vi "init.vi"(10 "WebBrowser":refnum<k7>(container), 11 "VI in":refnum<vi>) -> (0 "error out":errorcluster, 1 "Lab Description:":string, 2 "solution":dbl, 3 "lab":dbl)   [LabVIEW 2014]
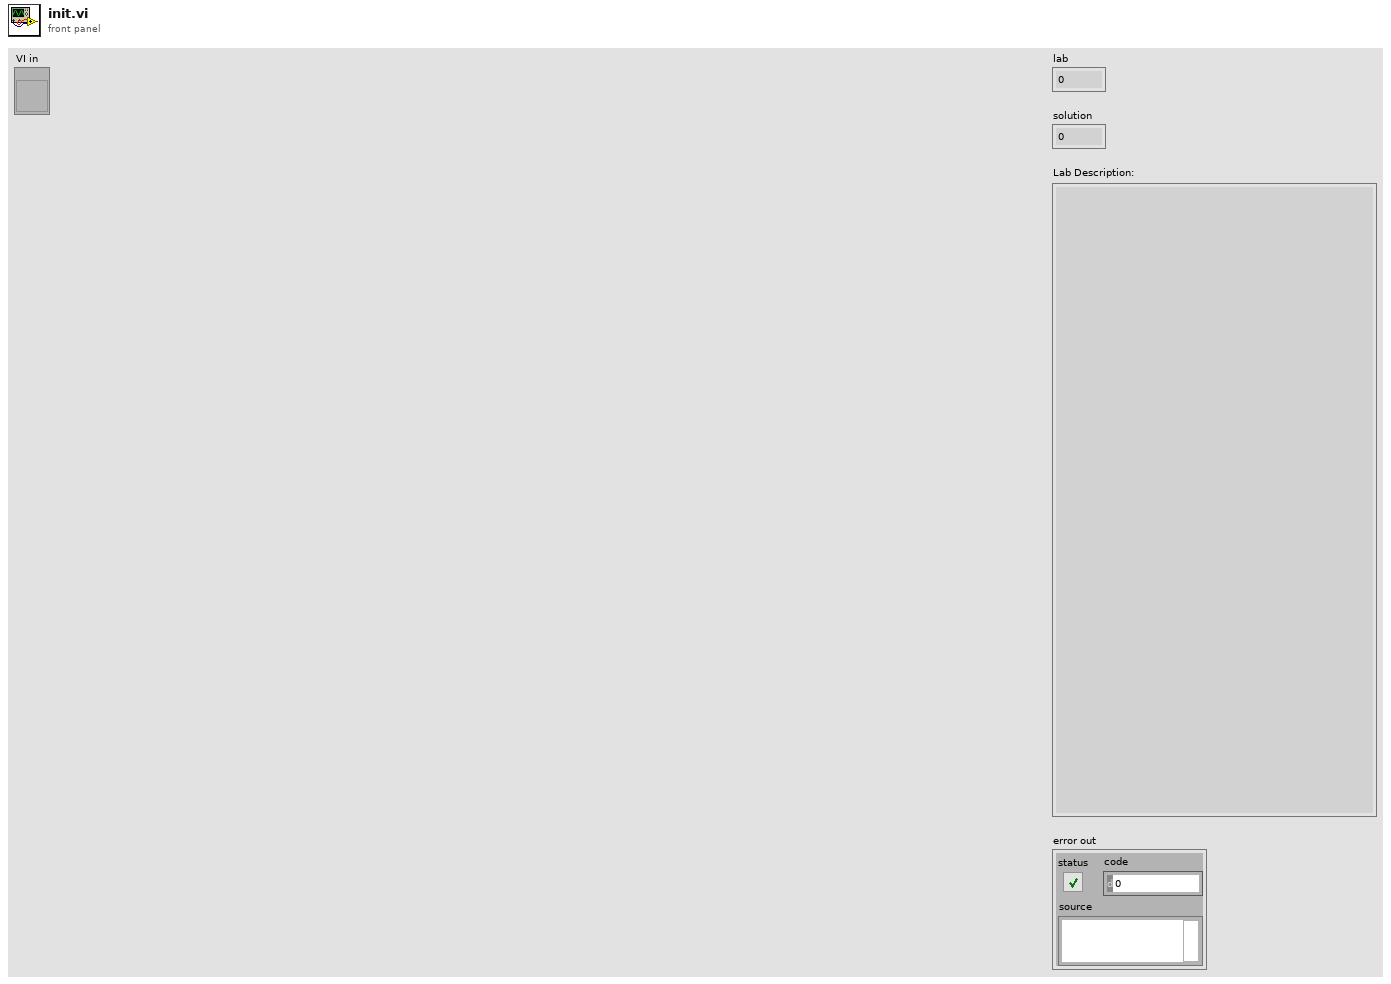
[diagram p1: front panel]
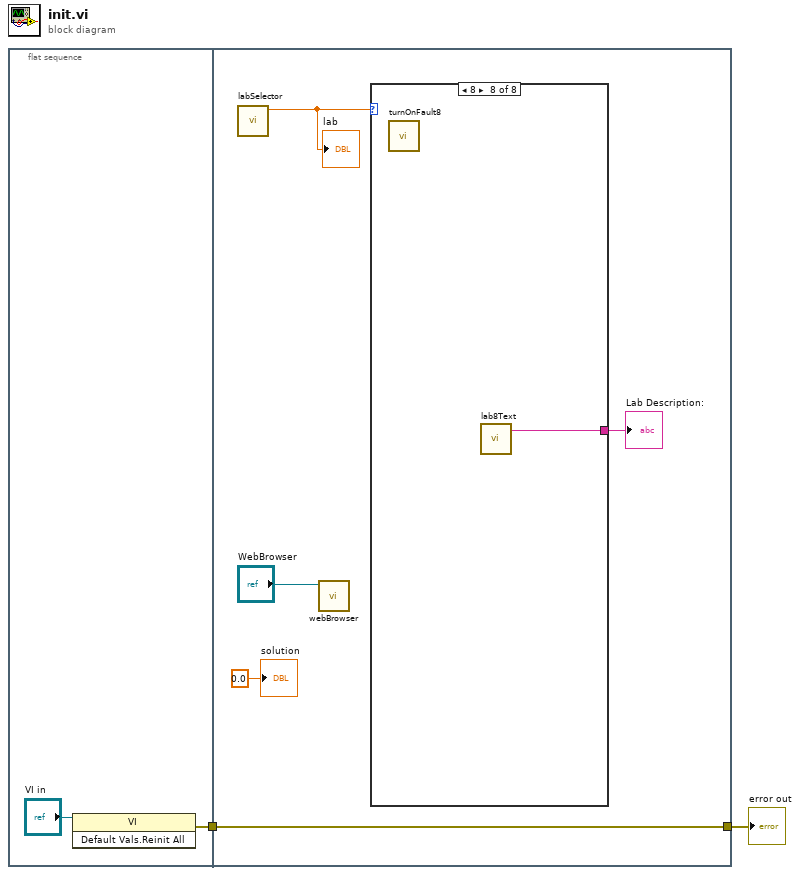
[diagram p0: block diagram]
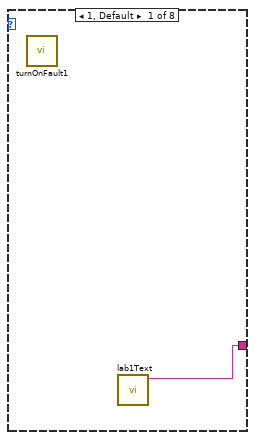
[diagram p2: hidden frame]
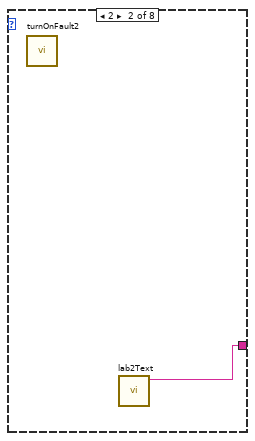
[diagram p3: hidden frame]
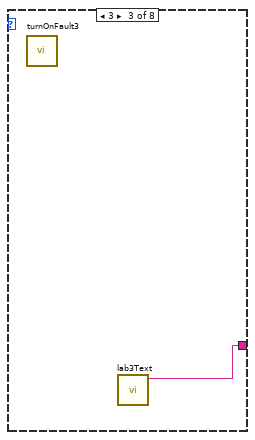
[diagram p4: hidden frame]
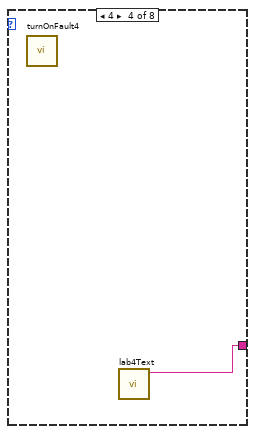
[diagram p5: hidden frame]
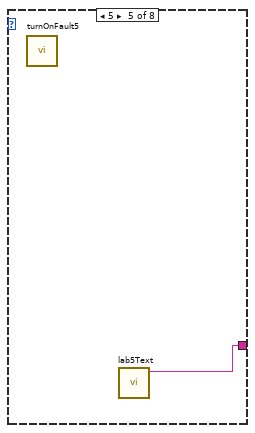
[diagram p6: hidden frame]
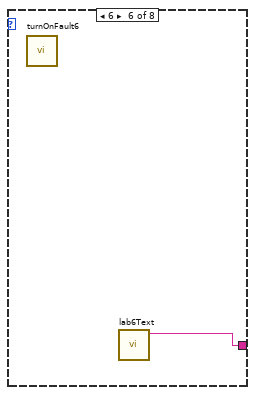
[diagram p7: hidden frame]
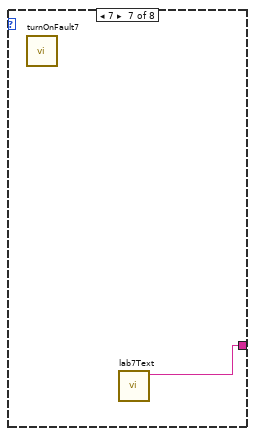
[diagram p8: hidden frame]
diagram:
  n1 = flat-sequence {
    tunnel: [w3] -> w2
    tunnel: w2 -> [w6]
    tunnel: [w6] -> w1
    frame #0 {
      n2 = invoke class="VI" method="Default Vals.Reinit All"(reference="VI in") -> (error out=w3:errorcluster)  [unwired: 2 in, 2 out]
    }
    frame #1 {
      n3 = call "labSelector.vi"() -> ("Numeric"=w7:dbl)  [unwired: 11 in]
      "lab" <- w7
      n4 = call "webBrowser.vi"("Automation Refnum in"="WebBrowser") -> ()  [unwired: 11 in]
      n5 = case shown="8" w7 {
        tunnel: [w10 w11 w12 w13 w14 w15 w16 w17] -> w5
        frame 1, Default {
          n6 = call "turnOnFault1.vi"() -> ()  [unwired: 12 in]
          n7 = call "lab1Text.vi"() -> ("String"=w10:string)  [unwired: 11 in]
        }
        frame 2 {
          n8 = call "turnOnFault2.vi"() -> ()  [unwired: 12 in]
          n9 = call "lab2Text.vi"() -> ("String"=w11:string)  [unwired: 11 in]
        }
        frame 3 {
          n10 = call "turnOnFault3.vi"() -> ()  [unwired: 12 in]
          n11 = call "lab3Text.vi"() -> ("String"=w12:string)  [unwired: 11 in]
        }
        frame 4 {
          n12 = call "turnOnFault4.vi"() -> ()  [unwired: 12 in]
          n13 = call "lab4Text.vi"() -> ("String"=w13:string)  [unwired: 11 in]
        }
        frame 5 {
          n14 = call "turnOnFault5.vi"() -> ()  [unwired: 12 in]
          n15 = call "lab5Text.vi"() -> ("String"=w14:string)  [unwired: 11 in]
        }
        frame 6 {
          n16 = call "turnOnFault6.vi"() -> ()  [unwired: 12 in]
          n17 = call "lab6Text.vi"() -> ("String"=w15:string)  [unwired: 11 in]
        }
        frame 7 {
          n18 = call "turnOnFault7.vi"() -> ()  [unwired: 12 in]
          n19 = call "lab7Text.vi"() -> ("String"=w16:string)  [unwired: 11 in]
        }
        frame 8 {
          n20 = call "turnOnFault8.vi"() -> ()  [unwired: 12 in]
          n21 = call "lab8Text.vi"() -> ("String"=w17:string)  [unwired: 11 in]
        }
      }
      "Lab Description:" <- w5
      "solution" <- 0.0 ("Numeric")
    }
  }
  "error out" <- w1
